vi "Dictionary Test - 004.vi"(8 "error in (no error)":errorcluster) -> (0 "error out":errorcluster, 2 "pass":bool)   [LabVIEW 2009]
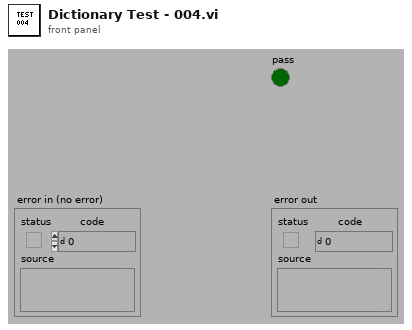
[diagram p1: front panel]
types:
  T1 = typedef "Dictionary Object RefNum.ctl" = refnum<k1>
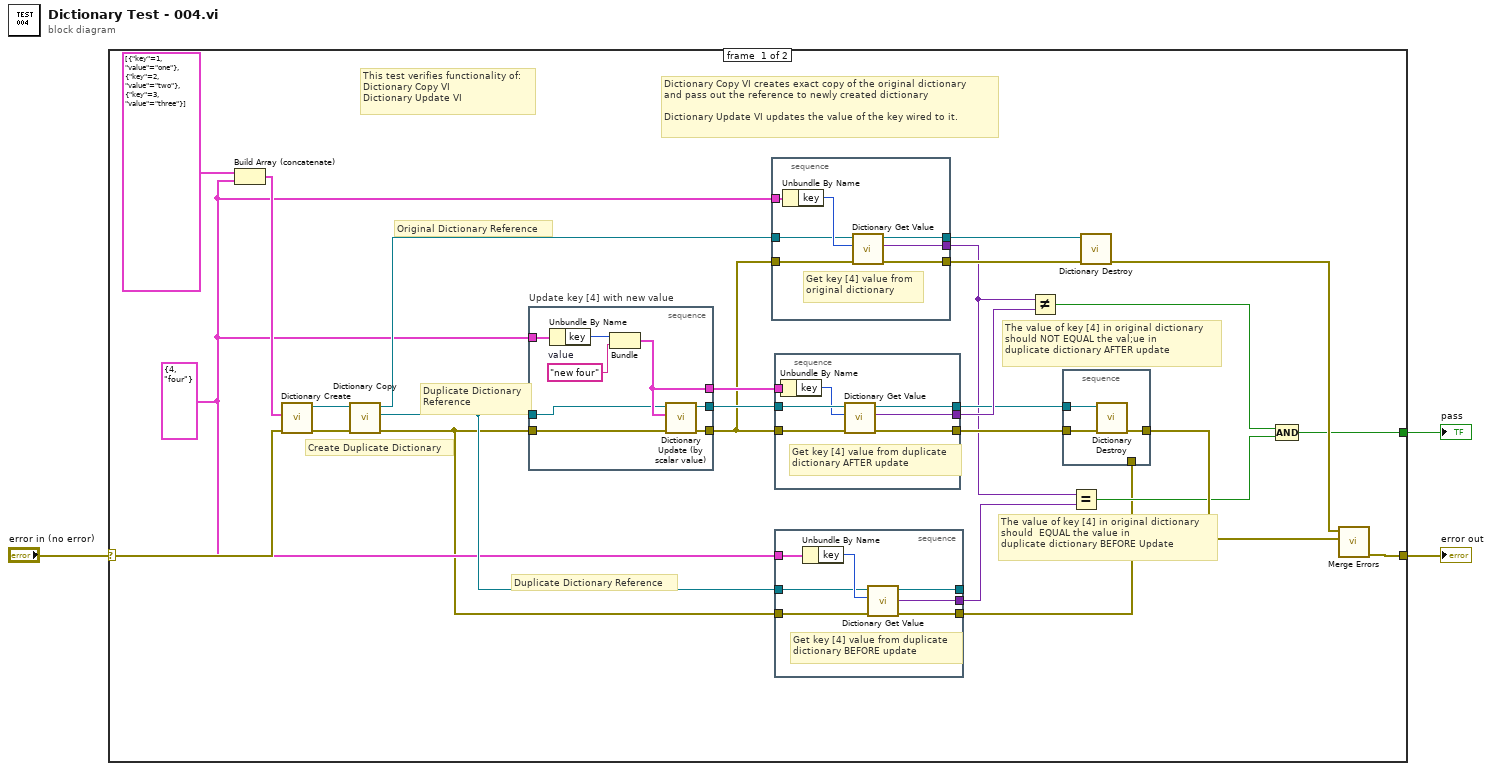
[diagram p0: block diagram]
diagram:
  n1 = case shown="No Error" "error in (no error)" {
    selector: "error in (no error)" -> [w29 w62]
    tunnel: [w18 w62] -> w2
    tunnel: [w8 _] -> w1
    frame #0 {
      w11 = cluster{"key":i32, "value":string} {"key"=4, "value"="four"}
      # "The value of key [4] in original dictionary\nshould  EQUAL the value in \nduplicate dictionary BEFORE Update"
      # "The value of key [4] in original dictionary\nshould NOT EQUAL the val;ue in \nduplicate dictionary AFTER update"
      # "Duplicate Dictionary Reference"
      # "Duplicate Dictionary\nReference"
      # "Original Dictionary Reference"
      # "Create Duplicate Dictionary"
      # "Dictionary Copy VI creates exact copy of the original dictionary \nand pass out the reference to newly created dictionary\n\nDictionary Update VI updates the value of the key wired to it."
      # "This test verifies functionality of:\nDictionary Copy VI\nDictionary Update VI"
      n2 = Build Array (concatenate)(cluster{"key":i32, "value":string}[] [{"key"=1, "value"="one"}, {"key"=2, "value"="two"}, {"key"=3, "value"="three"}] ("dictionary with updates"), w11) -> (w15:cluster{"key":i32, "value":string}[])
      n3 = call "Dictionary Create.vi"("error in (no error)"=w29, "initial dictionary (empty)"=w15) -> ("error out"=w26:errorcluster, "dictionary out"=w27:T1)  [unwired: 8 in]
      n4 = call "Dictionary Copy.vi"("error in (no error)"=w26, "dictionary"=w27) -> ("error out"=w5:errorcluster, "new dictionary out"=w12:T1, "dictionary out"=w13:T1)  [unwired: 7 in]
      n5 = stacked-sequence "Update key [4] with new value" {
        tunnel: [w61] -> w25
        tunnel: [w60] -> w24
        tunnel: w12 -> [w57]
        tunnel: w11 -> [w56]
        tunnel: [w55] -> w6
        tunnel: w5 -> [w54]
        frame #0 {
          w58 = "new four"  # value
          n6 = Unbundle By Name(w56) -> ("key"=w59:i32)
          n7 = Bundle("key"=w59, "value"=w58) -> (w60:cluster{"key":i32, "value":string})  [unwired: 1 in]
          n8 = call "Dictionary Update (by scalar value).vi"("error in (no error)"=w54, "key-value"=w60, "dictionary"=w57) -> ("error out"=w55:errorcluster, "dictionary out"=w61:T1)  [unwired: 6 in, 1 out]
        }
      }
      n9 = stacked-sequence {
        tunnel: [w53] -> w21
        tunnel: [w52] -> w19
        tunnel: w13 -> [w50]
        tunnel: w11 -> [w49]
        tunnel: [w48] -> w9
        tunnel: w6 -> [w47]
        frame #0 {
          # "Get key [4] value from\noriginal dictionary"
          n10 = Unbundle By Name(w49) -> ("key"=w51:i32)
          n11 = call "Dictionary Get Value.vi"("error in"=w47, "key"=w51, "dictionary"=w50) -> ("error out"=w52:errorcluster, "value"=w48:variant, "dictionary out"=w53:T1)  [unwired: 5 in, 1 out]
        }
      }
      n12 = stacked-sequence {
        tunnel: w25 -> [w46]
        tunnel: w24 -> [w45]
        tunnel: [w44] -> w23
        tunnel: [w43] -> w22
        tunnel: [w42] -> w20
        tunnel: w6 -> [w40]
        frame #0 {
          # "Get key [4] value from duplicate\ndictionary AFTER update"
          n13 = Unbundle By Name(w45) -> ("key"=w41:i32)
          n14 = call "Dictionary Get Value.vi"("error in"=w40, "key"=w41, "dictionary"=w46) -> ("error out"=w42:errorcluster, "value"=w44:variant, "dictionary out"=w43:T1)  [unwired: 5 in, 1 out]
        }
      }
      n15 = stacked-sequence {
        tunnel: w12 -> [w38]
        tunnel: w11 -> [w37]
        tunnel: [w36] -> w4
        tunnel: [w35] -> w10
        tunnel: w5 -> [w34]
        tunnel: [w33] -> _
        frame #0 {
          # "Get key [4] value from duplicate\ndictionary BEFORE update"
          n16 = Unbundle By Name(w37) -> ("key"=w39:i32)
          n17 = call "Dictionary Get Value.vi"("error in"=w34, "key"=w39, "dictionary"=w38) -> ("error out"=w36:errorcluster, "value"=w35:variant, "dictionary out"=w33:T1)  [unwired: 5 in, 1 out]
        }
      }
      n18 = Not Equal?(x=w9, y=w23) -> (x != y?=w14:bool)
      n19 = stacked-sequence {
        tunnel: w22 -> [w32]
        tunnel: w20 -> [w31]
        tunnel: [w30] -> w16
        tunnel: w4 -> [_]
        frame #0 {
          n20 = call "Dictionary Destroy.vi"("error in (no error)"=w31, "dictionary"=w32) -> ("error out"=w30:errorcluster)  [unwired: 9 in]
        }
      }
      n21 = Equal?(x=w9, y=w10) -> (x = y?=w7:bool)
      n22 = call "Dictionary Destroy.vi"("error in (no error)"=w19, "dictionary"=w21) -> ("error out"=w17:errorcluster)  [unwired: 9 in]
      n23 = Compound Arithmetic op=AND(w14, w7) -> (w8:bool)
      n24 = call <vilib>:"Merge Errors.vi"("error in 2 (no error)"=w16, "error in 1 (no error)"=w17) -> ("error out"=w18:errorcluster)  [unwired: 5 in]
    }
    frame #1 {
    }
  }
  "pass" <- w1
  "error out" <- w2
